vi "loadData.vi"(2 "error in (no error)":errorcluster, 3 "Data":dbl[][](array[numeric]), 4 "AnalogOutput in":refnum<class "AnalogOutput.lvclass">) -> (0 "error out":errorcluster, 1 "AnalogOutput out":refnum<class "AnalogOutput.lvclass">)   [LabVIEW 2011, in "Hardware.lvlib" / "Channels.lvlib" / "AnalogOutput.lvclass"]
doc: "Abstract Method.\n\nThis vi first stores the passed data for the analog output and then calls loadDataToBuffer.vi to actually load the data into the hardware devices buffer. loadDataToBuffer.vi is implemeted by child classes.\n\nCluster passed:\n1) Data (1D Array of Waveform(DBL), one waveform per channel)"
uses:
  AnalogOutput.lvclass
  AnalogOutput.lvclass/AnalogOutput.ctl
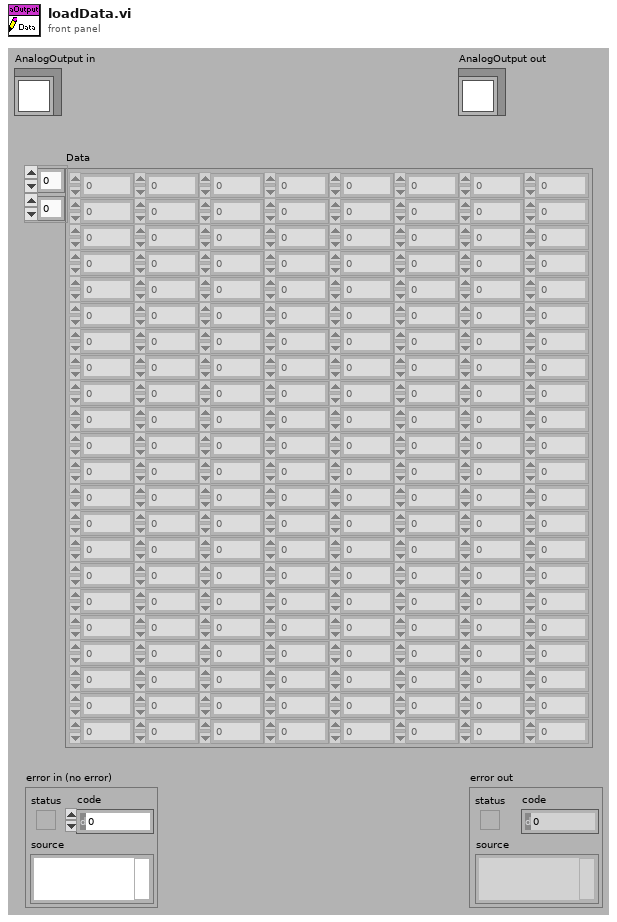
[diagram p1: front panel]
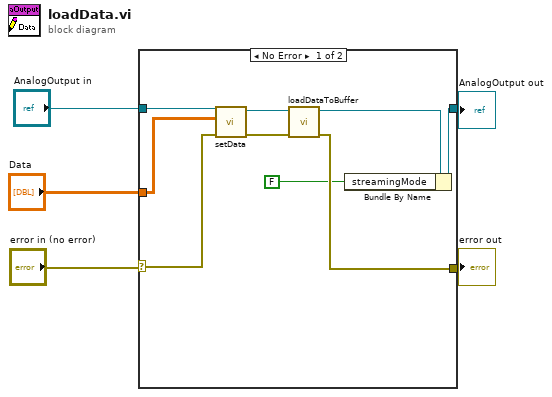
[diagram p0: block diagram]
diagram:
  n1 = case shown="No Error" "error in (no error)" {
    selector: "error in (no error)" -> [w13 w16]
    tunnel: [w10 w16] -> w4
    tunnel: [w6 w15] -> w2
    tunnel: "AnalogOutput in" -> [w14 w15]
    tunnel: "Data" -> [w9 _]
    frame No Error {
      n2 = call "setData.vi"("error in (no error)"=w13, "Data"=w9, "AnalogOutput.lvclass in"=w14) -> ("error out"=w11:errorcluster, "AnalogOutput.lvclass out"=w12:refnum<class "AnalogOutput.lvclass">)  [unwired: 7 in]
      n3 = call-dynamic "loadDataToBuffer.vi"("error in (no error)"=w11, "AnalogOutput in"=w12) -> ("error out"=w10:errorcluster, "AnalogOutput out"=w7:refnum<class "AnalogOutput.lvclass">)  [unwired: 8 in]
      n4 = Bundle By Name(cluster=w7, "streamingMode"=FALSE) -> (w6:refnum<class "AnalogOutput.lvclass">)
    }
    frame Error {
    }
  }
  "error out" <- w4
  "AnalogOutput out" <- w2
